vi "Initialize Globals.vi"(5 "Abort Refnum":refnum<vi>, 7 "Status Refnum":refnum<vi>, 8 "error in (pass through)":errorcluster, 9 "Debug mode":T1, 10 "Timeouts":T2={"TCP Read & Write (ms)"=7000, "Sensors readout"=5000, "PJVS setup"=10000, "Nullmeter readout"=5000, "Multiplexer setup"=3000, "57XX setup"=15000, "Generator setup"=5000, "Synthesizer setup"=3000, "Sampler readout"=10000}, 11 "IP address:port (0.0.0.0:0000)":string="0.0.0.0:0000") -> (0 "error out":errorcluster, 1 "Debug mode out":T1, 2 "Timeouts out":T2={"TCP Read & Write (ms)"=7000, "Sensors readout"=5000, "PJVS setup"=5000, "Nullmeter readout"=5000, "Multiplexer setup"=3000, "57XX setup"=5000, "Generator setup"=5000, "Synthesizer setup"=3000, "Sampler readout"=10000}, 3 "IP address:port out":string, 4 "Abort Refnum out":refnum<vi>, 6 "Status Refnum out":refnum<vi>)   [LabVIEW 2019, in "ACSVcontrol-driver.lvlib"]
doc: "Initializes the PJVS driver. Sets IP address of the PJVS control computer, sets timeouts and refnum to status field and abort button.\n\nAll unwired inputs retains the values from previous setting. If only IP address have to be changed, wire only this input, etc.\n\nAt the beginning at least IP address have to be set."
uses:
  ACSVcontrol-driver.lvlib
  Type Definitions/Timeouts.ctl
  Type Definitions/Debug status.ctl
  Private/Globals.vi
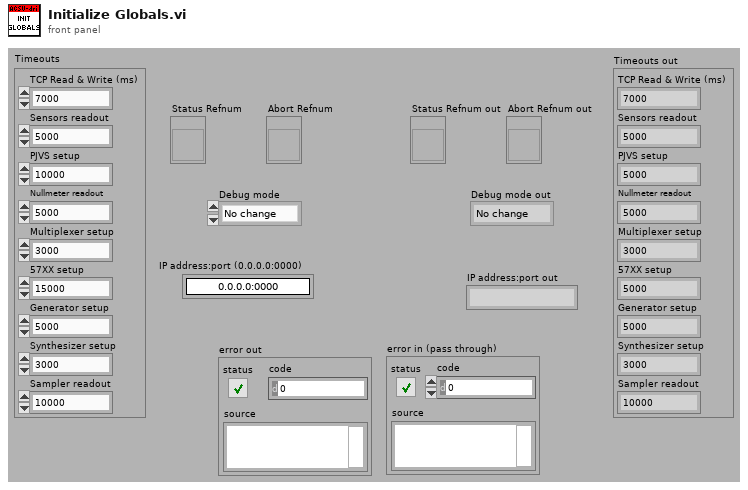
[diagram p1: front panel]
types:
  T1 = typedef "ACSVcontrol-driver.lvlib/Debug status.ctl" = enum16{"No change", "Off", "On"}
  T2 = typedef "ACSVcontrol-driver.lvlib/Timeouts.ctl" = cluster{"TCP Read & Write (ms)":i32, "Sensors readout":i32, "PJVS setup":i32, "Nullmeter readout":i32, "Multiplexer setup":i32, "57XX setup":i32, "Generator setup":i32, "Synthesizer setup":i32, "Sampler readout":i32}
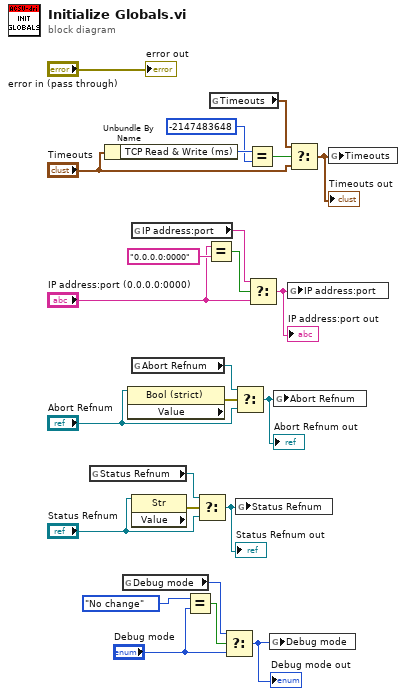
[diagram p0: block diagram]
diagram:
  n1 = global read "Globals.vi" "Status Refnum"() -> (w14:refnum<vi>)
  n2 = Unbundle By Name("Timeouts") -> ("TCP Read & Write (ms)"=w25:i32)
  n3 = global read "Globals.vi" "Debug mode"() -> (w3:T1)
  n4 = property class="Bool (strict)" props=["Value"](reference="Abort Refnum") -> (error out=w11:errorcluster)  [unwired: 1 in, 2 out]
  n5 = global read "Globals.vi" "IP address:port"() -> (w17:string)
  n6 = global read "Globals.vi" "Abort Refnum"() -> (w9:refnum<vi>)
  n7 = property class="Str" props=["Value"](reference="Status Refnum") -> (error out=w6:errorcluster)  [unwired: 1 in, 2 out]
  n8 = Equal?(x=Debug_status."No change" ("y"), y="Debug mode") -> (x = y?=w4:bool)
  n9 = Select(t=w14, s=w6, f="Status Refnum") -> (s? t:f=w13:refnum<vi>)
  "Status Refnum out" <- w13
  n10 = Equal?(x="IP address:port (0.0.0.0:0000)", y="0.0.0.0:0000") -> (x = y?=w16:bool)
  n11 = global read "Globals.vi" "Timeouts"() -> (w22:T2)
  n12 = Select(t=w3, s=w4, f="Debug mode") -> (s? t:f=w1:T1)
  "Debug mode out" <- w1
  n13 = Select(t=w9, s=w11, f="Abort Refnum") -> (s? t:f=w10:refnum<vi>)
  "Abort Refnum out" <- w10
  n14 = global write "Globals.vi" "Status Refnum"(w13) -> ()
  n15 = Equal?(x=w25, y=-2147483648) -> (x = y?=w23:bool)
  n16 = Select(t=w17, s=w16, f="IP address:port (0.0.0.0:0000)") -> (s? t:f=w18:string)
  "IP address:port out" <- w18
  n17 = global write "Globals.vi" "Debug mode"(w1) -> ()
  n18 = global write "Globals.vi" "Abort Refnum"(w10) -> ()
  n19 = global write "Globals.vi" "IP address:port"(w18) -> ()
  n20 = Select(t=w22, s=w23, f="Timeouts") -> (s? t:f=w21:T2)
  "Timeouts out" <- w21
  n21 = global write "Globals.vi" "Timeouts"(w21) -> ()
  "error out" <- "error in (pass through)"
